vi "calcOpt.vi"() -> (2 "Optical State":dbl[](array[numeric]))   [LabVIEW 2016]
uses:
  OptStateEsti/OptStateEsti.lvclass
  StrictDef/InstName.ctl
  <vilib>/Analysis/baseanly.llb/Real A x B.vi
  <vilib>/Analysis/Matrix/Numeric/Conversions/Array To Matrix - RA2.vi
  <vilib>/Analysis/Matrix/Numeric/Conversions/Array To Matrix - RA.vi
  <vilib>/Analysis/Matrix/Numeric/Conversions/Matrix To Array - RM.vi
  <vilib>/Analysis/Matrix/NI_Matrix.lvlib
  <vilib>/Analysis/NI_AALBase.lvlib
panel:
  in  "Configuration":T2={"Config Dir"=path "/home/ttsai/Documents/stash/ts_tcs_ofc/configData", "Inst Name"=enum."lsst", "Config File Name"="pinv.esti", "Mapping File Name"="sensorNameToFieldIdx.txt", "Wavelength Table"="effWaveLength.txt", "Intrinc Zk File Name"="intrinsic_zn"}
  out "Array":dbl[][](array[numeric])
  out "output array":dbl[][](array[numeric])
  out "XY Graph":cluster{"Idx Array":i32[], dbl[]}[](graph)
  out "WFS Err":dbl[][](array[numeric])
  out "size(s) 3":i32[](array[numeric])
  in  "Wfs Err Data":path=path "/home/ttsai/Documents/stash/ts_tcs_ofc/testData/sim6_iter0_E000.z4c"
  in  "Sen M File Name":string="senM_35_19_50.txt"
  in  "Sensor Name":string[](array[string])=["R:4,4 S:0,0", "R:0,4 S:2,0", "R:0,0 S:2,2", "R:4,0 S:0,2"]
  out "size(s) 2":i32[](array[numeric])
  out "Pinv A":dbl[][](array[numeric])
  in  "Truncation Threshold":dbl=0.0001
  out "Stacked 2D Array":dbl[][](array[numeric])
  out "Field Idx":i32[](array[numeric])
  out "size(s)":i32[](array[numeric])
  out "Sen M":dbl[][][](array[numeric])
  in  "OptStateEsti in":refnum<class "OptStateEsti.lvclass">
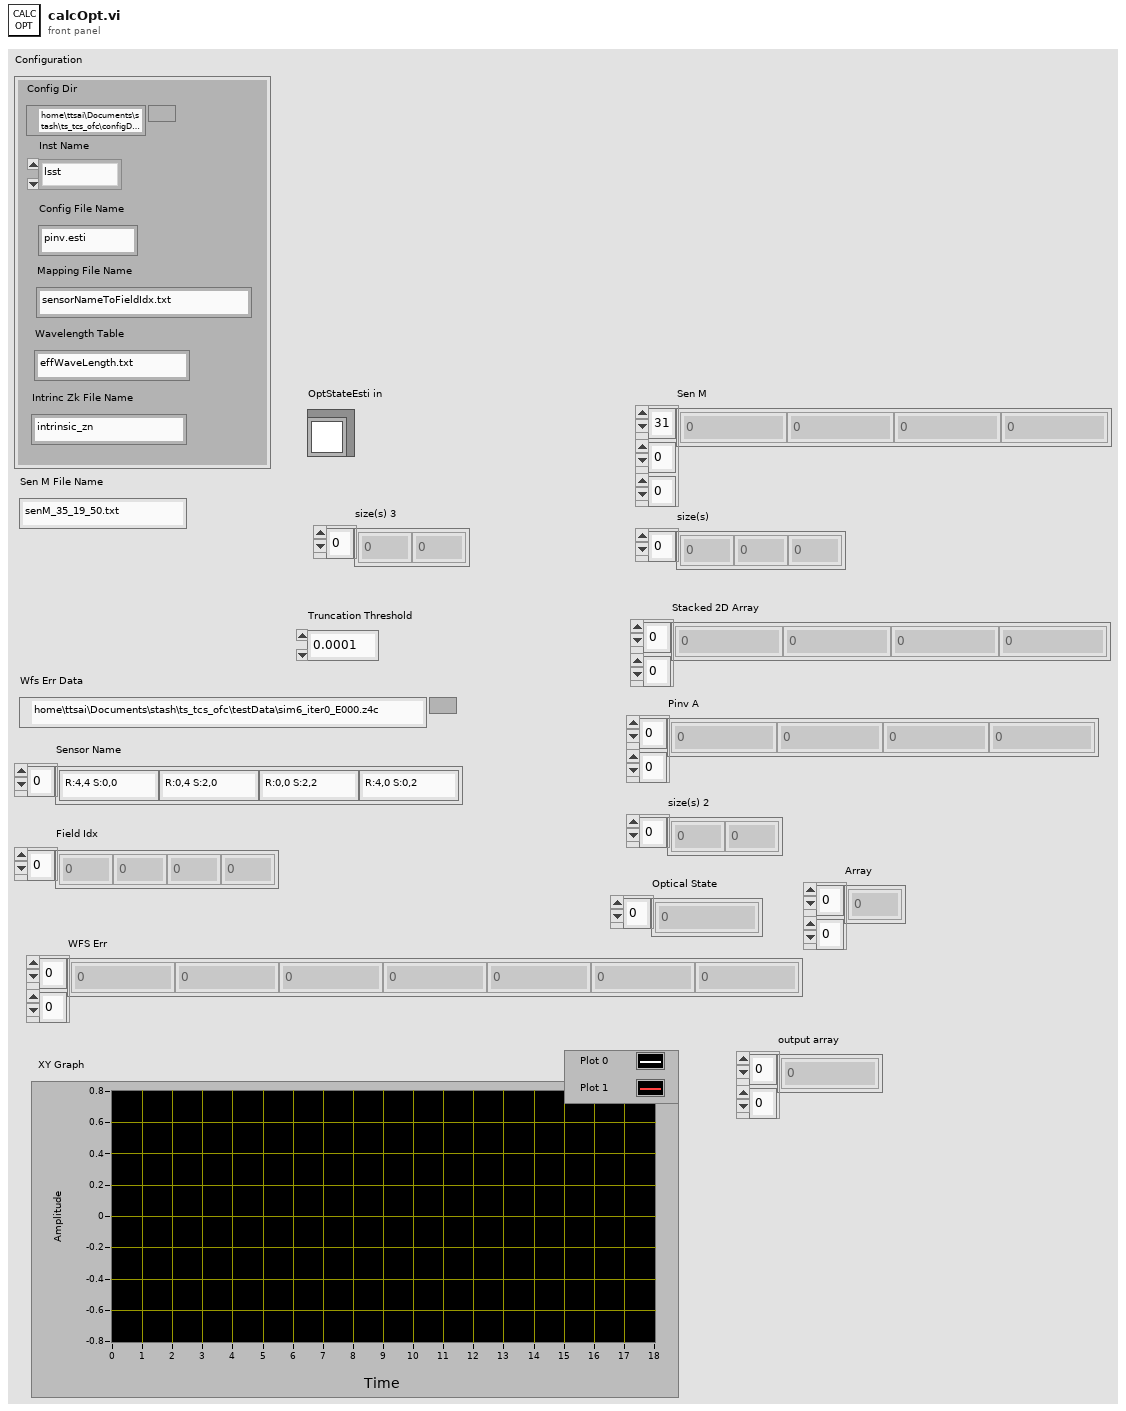
[diagram p1: front panel]
types:
  T1 = typedef "InstName.ctl" = enum16{"lsst", "comcam"}
  T2 = cluster{"Config Dir":path, "Inst Name":T1, "Config File Name":string, "Mapping File Name":string, "Wavelength Table":string, "Intrinc Zk File Name":string}
  T3 = typedef "NI_Matrix.lvlib/RealMatrix.ctl" = dbl[][]
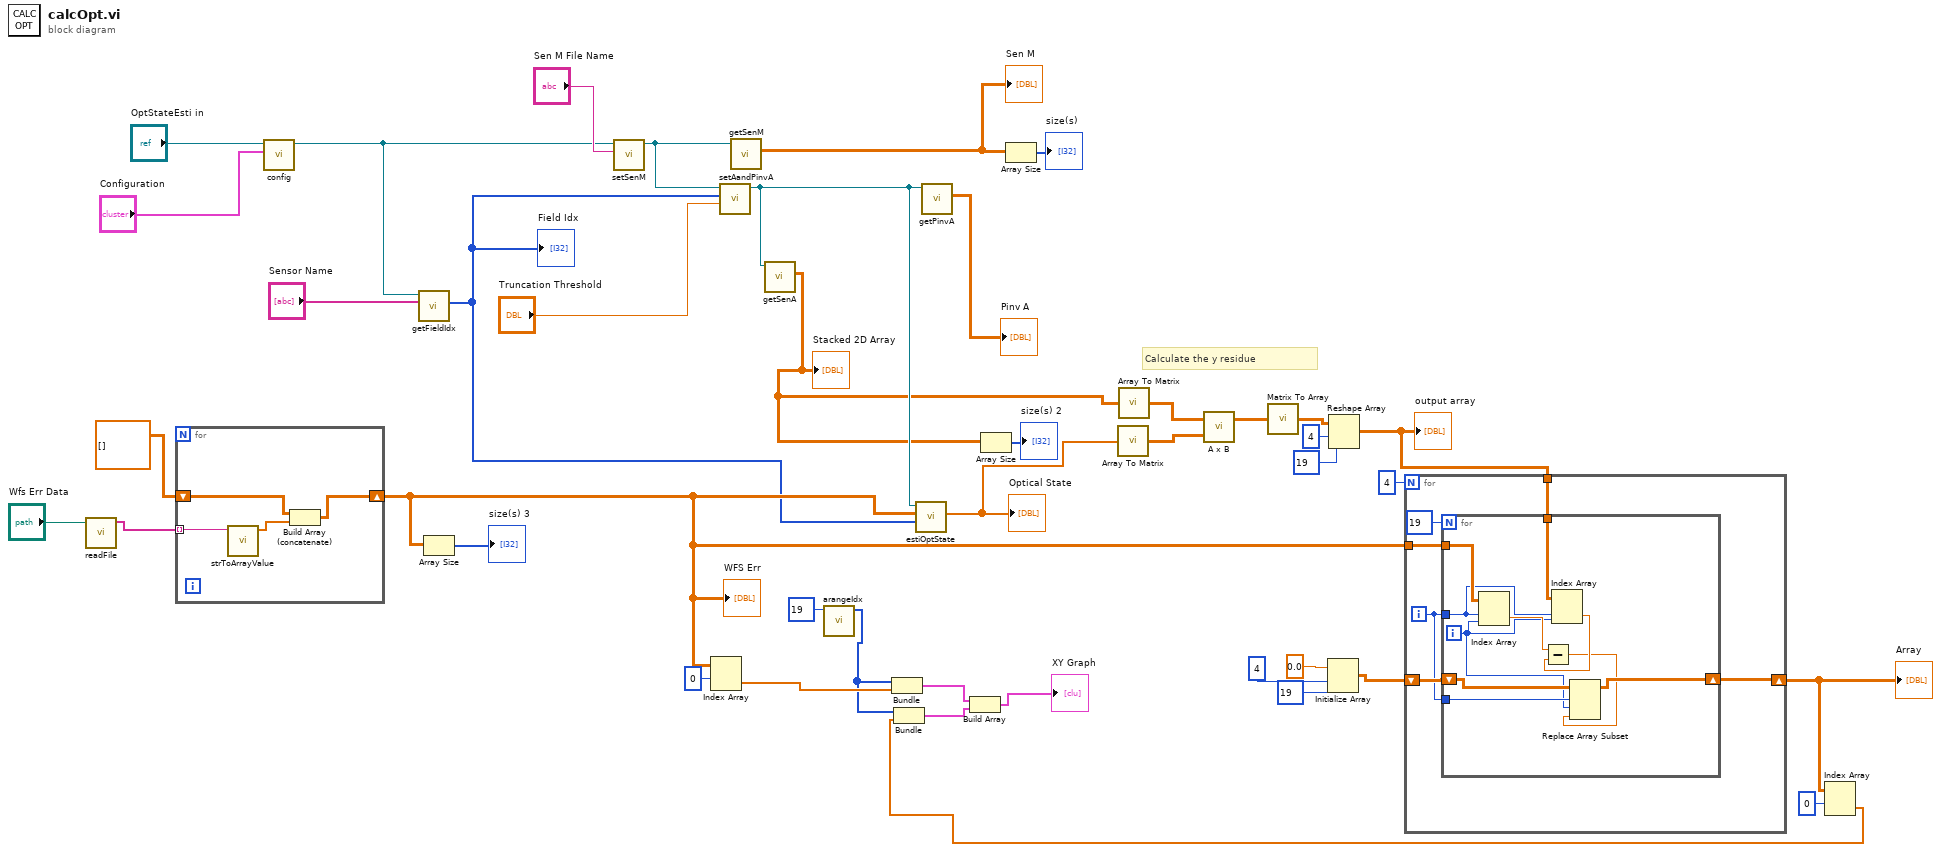
[diagram p0: block diagram]
diagram:
  # "Calculate the y residue"
  n1 = call "readFile.vi"("Path"="Wfs Err Data") -> ("Array"=w35:string[])  [unwired: 9 in, 1 out]
  n2 = for {
    shift-right: [w43] -> w14
    shift-left: dbl[][] [] -> [w44]
    tunnel: w35 -> [w46] mode=indexing
    n3 = call "strToArrayValue.vi"("String"=w46) -> ("Array"=w45:dbl[])  [unwired: 9 in, 1 out]
    n4 = Build Array (concatenate)(w44, w45) -> (w43:dbl[][])
  }
  "WFS Err" <- w14
  n5 = call "config.vi"("Configuration"="Configuration", "OptStateEsti in"="OptStateEsti in") -> ("OptStateEsti out"=w8:refnum<class "OptStateEsti.lvclass">)  [unwired: 8 in, 1 out]
  n6 = call "getFieldIdx.vi"("Sensor Name"="Sensor Name", "OptStateEsti in"=w8) -> ("Field Idx"=w5:i32[])  [unwired: 7 in, 2 out]
  "Field Idx" <- w5
  n7 = Array Size(array=w14) -> (size(s)=→"size(s) 3":i32[])
  n8 = call "setSenM.vi"("Sen M File Name"="Sen M File Name", "OptStateEsti in"=w8) -> ("OptStateEsti out"=w6:refnum<class "OptStateEsti.lvclass">)  [unwired: 8 in, 1 out]
  n9 = Index Array(array=w14, index (row)=0) -> (element=w30:dbl[])  [unwired: 1 in]
  n10 = call "setAandPinvA.vi"("Truncation Threshold"="Truncation Threshold", "Field Idx"=w5, "OptStateEsti in"=w6) -> ("OptStateEsti out"=w3:refnum<class "OptStateEsti.lvclass">)  [unwired: 7 in, 1 out]
  n11 = call "getSenM.vi"("OptStateEsti in"=w6) -> ("Sen M"=w41:dbl[][][])  [unwired: 8 in, 2 out]
  "Sen M" <- w41
  n12 = call "getSenA.vi"("OptStateEsti in"=w3) -> ("Matrix A"=w2:dbl[][])  [unwired: 8 in, 2 out]
  "Stacked 2D Array" <- w2
  n13 = call "arangeIdx.vi"("Number"=19) -> ("Idx Array"=w29:i32[])  [unwired: 10 in]
  n14 = Bundle("Idx Array"=w29, w30) -> (w28:cluster{"Idx Array":i32[], dbl[]})  [unwired: 1 in]
  n15 = call "estiOptState.vi"("Field Idx"=w5, "Zk"=w14, "OptStateEsti in"=w3) -> ("Optical State"=w25:dbl[])  [unwired: 6 in, 2 out]
  "Optical State" <- w25
  n16 = call "getPinvA.vi"("OptStateEsti in"=w3) -> ("Pinv A"=→"Pinv A":dbl[][])  [unwired: 8 in, 2 out]
  n17 = Array Size(array=w2) -> (size(s)=→"size(s) 2":i32[])
  n18 = Array Size(array=w41) -> (size(s)=→"size(s)":i32[])
  n19 = call-poly <vilib>:"Array To Matrix.vi"("Real 1D Array"=w25) -> ("Real Matrix (Column Vector)"=w23:T3)
  n20 = call-poly <vilib>:"Array To Matrix.vi"("Real 2D Array"=w2) -> ("Real Matrix"=w24:T3)
  n21 = call-poly <vilib>:"A x B.vi"("B"=w23, "A"=w24) -> ("A x B"=w22:T3)  [unwired: 1 out]
  n22 = call-poly <vilib>:"Matrix To Array.vi"("Real Matrix"=w22) -> ("Real 2D Array"=w21:dbl[][])
  n23 = Initialize Array(0.0 ("element"), 4 ("dimension size"), 19 ("dimension size")) -> (w15:dbl[][])
  n24 = Reshape Array(w21, 4 ("dimension size"), 19 ("dimension size")) -> (w13:dbl[][])
  "output array" <- w13
  n25 = for {
    N: 4 -> [_]
    shift-right: [w51] -> w11
    shift-left: w15 -> [w52]
    tunnel: w14 -> [w50]
    tunnel: w13 -> [w49]
    i -> [w48]
    n26 = for {
      N: 19 -> [_]
      shift-right: [w56] -> w51
      shift-left: w52 -> [w57]
      tunnel: w48 -> [w61]
      tunnel: w50 -> [w62]
      tunnel: w49 -> [w60]
      tunnel: w48 -> [w55]
      i -> [w54]
      n27 = Index Array(array=w62, index (row)=w61, index (col)=w54) -> (element=w59:dbl)
      n28 = Index Array(array=w60, index (row)=w61, index (col)=w54) -> (element=w58:dbl)
      n29 = Subtract(x=w59, y=w58) -> (x-y=w53:dbl)
      n30 = Replace Array Subset(array=w57, new element=w53, index (row)=w55, index (col)=w54) -> (w56:dbl[][])
    }
  }
  "Array" <- w11
  n31 = Index Array(array=w11, index (row)=0) -> (element=w9:dbl[])  [unwired: 1 in]
  n32 = Bundle("Idx Array"=w29, w9) -> (w27:cluster{"Idx Array":i32[], dbl[]})  [unwired: 1 in]
  n33 = Build Array(w28, w27) -> (→"XY Graph":cluster{"Idx Array":i32[], dbl[]}[])
